vi "get.frame-name-from-tag.vi"(4 "tag":string) -> (1 "frame.name":string)   [LabVIEW 2015]
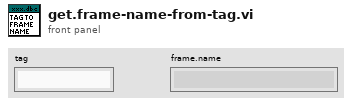
[diagram p1: front panel]
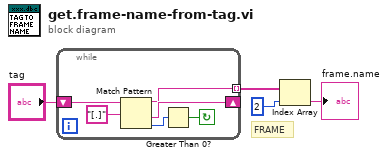
[diagram p0: block diagram]
diagram:
  # "FRAME"
  n1 = while {
    shift-right: [w9] -> _
    shift-left: "tag" -> [w10]
    tunnel: [w6] -> w3 mode=indexing
    stop <- w7 continue-if-true
    n2 = Match Pattern(string=w10, regular expression="[.]") -> (before substring=w6:string, after substring=w9:string, offset past match=w8:i32)  [unwired: 1 in, 1 out]
    n3 = Greater Than 0?(x=w8) -> (x > 0?=w7:bool)
  }
  n4 = Index Array(array=w3, index=2) -> (element=→"frame.name":string)
